vi "Convert to padded Trial number index string.vi"(11 "Trial number (unity-based)":i32=3) -> (2 "Trial number string padded with zeroes":string)   [LabVIEW 2017]
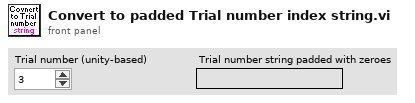
[diagram p1: front panel]
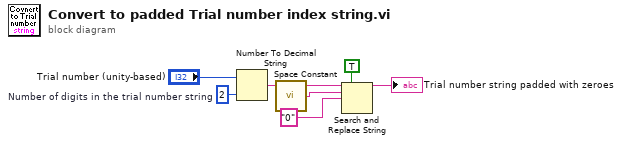
[diagram p0: block diagram]
diagram:
  w7 = i16 2  # Number of digits in the trial number string
  n1 = Number To Decimal String(number="Trial number (unity-based)", width (-)=w7) -> (decimal integer string=w5:string)
  n2 = call <vilib>:"Space Constant.vi"() -> ("String"=w2:string)
  n3 = Search and Replace String(replace all?=TRUE ("replace all? (F)"), input string=w5, search string=w2, replace string="0") -> (result string=→"Trial number string padded with zeroes":string)  [unwired: 4 in, 3 out]
